vi "Latch Boolean True.vi"(0 "Input":bool, 1 "Reset?":bool) -> (2 "Latched True":bool)   [LabVIEW 2013]
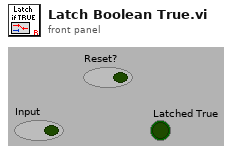
[diagram p1: front panel]
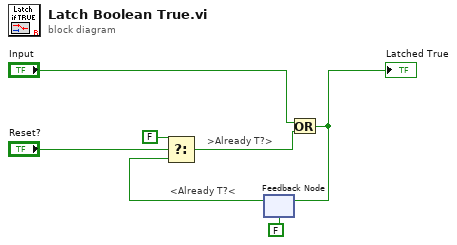
[diagram p0: block diagram]
diagram:
  # ">Already T?>"
  # "<Already T?<"
  n1 = feedback #1(FALSE) -> (w1:bool)
  n2 = Select(t=FALSE, s="Reset?", f=w1) -> (s? t:f=w5:bool)
  n3 = Or(x="Input", y=w5) -> (x .or. y?=w4:bool)
  "Latched True" <- w4
  n4 = feedback-in #1(w4) -> ()
